vi "Dialog_Initial.vi"(8 "error in":errorcluster, 11 "reference":refnum<vi>) -> (0 "error out":errorcluster)   [LabVIEW 2011]
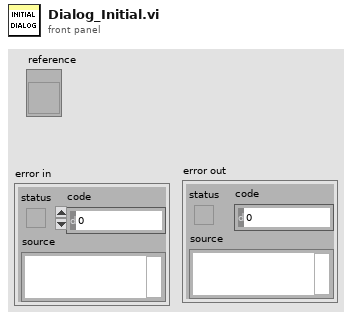
[diagram p1: front panel]
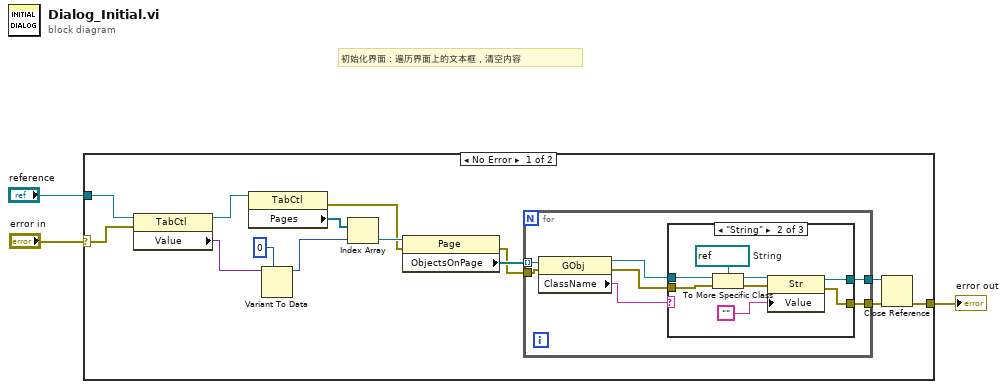
[diagram p0: block diagram]
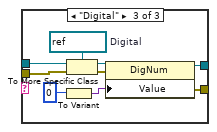
[diagram p3: hidden frame]
diagram:
  # "初始化界面：遍历界面上的文本框，清空内容"
  n1 = case shown="No Error" "error in" {
    selector: "error in" -> [w7 w44]
    tunnel: [w15 w44] -> w3
    tunnel: "reference" -> [w14 _]
    frame No Error {
      n2 = property class="TabCtl"(reference=w14, error in=w7) -> (reference out=w8:refnum<vi>, "Value"=w5:variant)  [unwired: 1 out]
      n3 = property class="TabCtl"(reference=w8) -> (error out=w9:errorcluster, "Pages"=w11:refnum<vi>[])  [unwired: 1 in, 1 out]
      n4 = Variant To Data(type=0, Variant=w5) -> (data=w4:i32)  [unwired: 1 in, 1 out]
      n5 = Index Array(array=w11, index=w4) -> (element=w10:refnum<vi>)
      n6 = property class="Page"(reference=w10, error in=w9) -> (error out=w12:errorcluster, "ObjectsOnPage"=w13:refnum<vi>[])  [unwired: 1 out]
      n7 = for {
        tunnel: w13 -> [w24] mode=indexing
        tunnel: w12 -> [w21]
        tunnel: [w20] -> w17
        tunnel: [w19] -> w16
        n8 = property class="GObj"(reference=w24, error in=w21) -> (reference out=w23:refnum<vi>, error out=w22:errorcluster, "ClassName"=w18:string)
        n9 = case shown="\"String\"" w18 {
          tunnel: w23 -> [w26 w34 w43]
          tunnel: w22 -> [w25 w29 w39]
          tunnel: [w26 w28 w38] -> w20
          tunnel: [w25 w27 w37] -> w19
          frame Default {
          }
          frame "String" {
            w33 = refnum<vi> refnum  # String
            n10 = To More Specific Class(target class=w33, reference=w34, error in=w29) -> (specific class reference=w32:refnum<vi>, error out=w31:errorcluster)
            n11 = property class="Str"(reference=w32, error in=w31, "Value"="") -> (reference out=w28:refnum<vi>, error out=w27:errorcluster)
          }
          frame "Digital" {
            w42 = refnum<vi> refnum  # Digital
            n12 = To Variant(anything=0) -> (Variant=w35:variant)
            n13 = To More Specific Class(target class=w42, reference=w43, error in=w39) -> (specific class reference=w41:refnum<vi>, error out=w40:errorcluster)
            n14 = property class="DigNum"(reference=w41, error in=w40, "Value"=w35) -> (reference out=w38:refnum<vi>, error out=w37:errorcluster)
          }
        }
      }
      n15 = Close Reference(reference=w17, error in (no error)=w16) -> (error out=w15:errorcluster)
    }
    frame Error {
    }
  }
  "error out" <- w3
